vi "test.vi"() -> ()   [LabVIEW 2020]
uses:
  DataSocketCluster external.ctl
panel:
  in  "TimeOut Time (s)":dbl=30.0 format="%.2f"
  out "Response Initialise":string
  out "Response to Load bias parameters":string
  in  "Load bias parameters":bool
  out "Voltage at each step on PJVS curve":dbl[](array[numeric]) format="%#_16g"
  in  "Send AC":bool
  out "Response to SEND AC":string
  out "Return number of steps on PJVS curve":string
  out "Return time interval on PJVS step":string
  out "Frequency calculated (Hz)":dbl=100.0
  in  "Frequency (Hz)":dbl=100.0 format="%#_10g"
  in  "Amplitude (V)":string="1"
  in  "Steps on PJVS curve":u32=100
  out "Calculated time on PJVS step (smallest value is 17)":u32=100
  in  "Name of computer running Bias Source software":string="CZC105BD8M"
  in  "This machine (client)":string="localhost"
  out "error out":errorcluster {"code" format="%.0x"}
  in  "error in (no error)":errorcluster
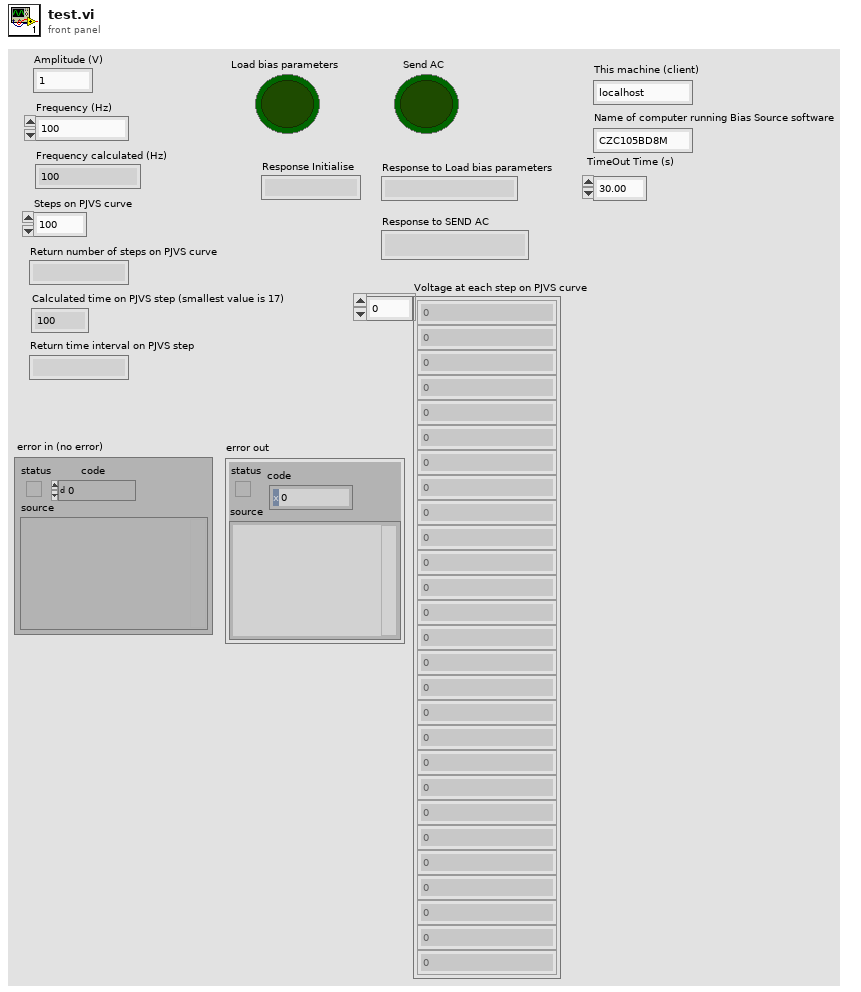
[diagram p1: front panel]
types:
  T1 = typedef "DataSocketCluster external.ctl" = cluster{"Server Machine":string, "Client Machine":string, "Data":string, "TimeStamp":dbl, "Count":i32, "Target Process":string}
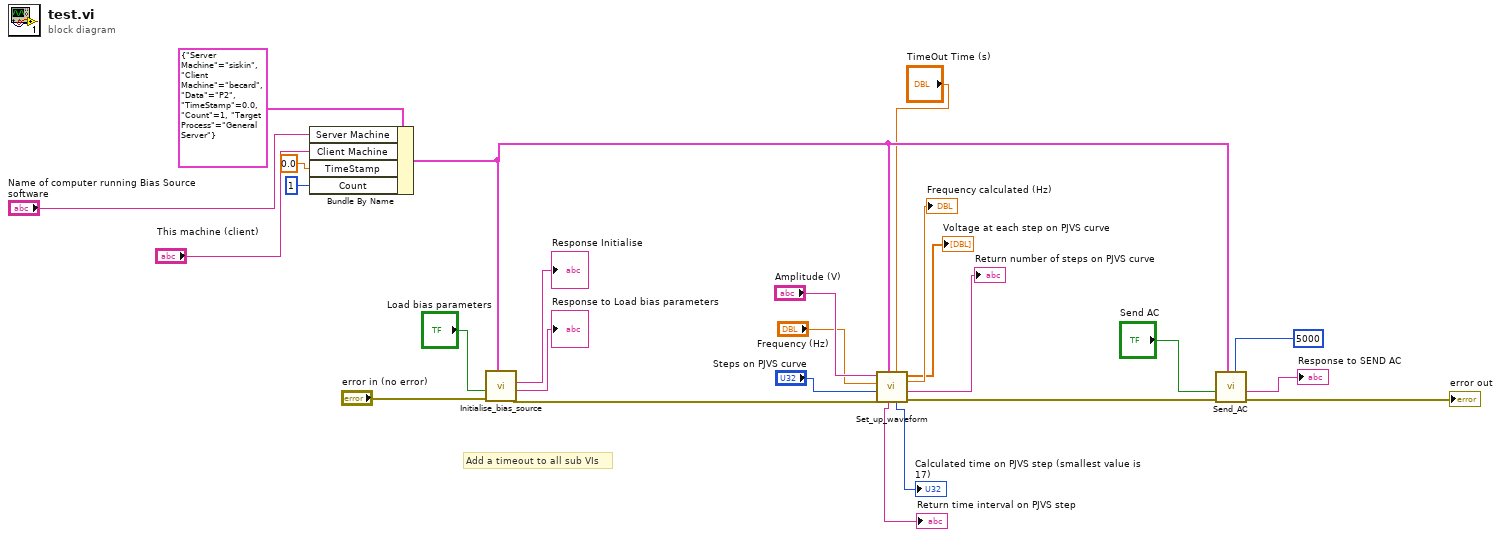
[diagram p0: block diagram]
diagram:
  # "Add a timeout to all sub VIs"
  n1 = Bundle By Name(cluster=T1 {"Server Machine"="siskin", "Client Machine"="becard", "Data"="P2", "TimeStamp"=0.0, "Count"=1, "Target Process"="General Server"} ("DataSocketCluster In"), "Server Machine"="Name of computer running Bias Source software", "Client Machine"="This machine (client)", "TimeStamp"=0.0, "Count"=1) -> (w5:T1)
  n2 = call "Initialise_bias_source.vi"("output cluster"=w5, "error in (no error)"="error in (no error)", "Load bias parameters"="Load bias parameters") -> ("error out"=w16:errorcluster, "Response to Load bias parameters"=→"Response to Load bias parameters":string, "Response Initialise"=→"Response Initialise":string)  [unwired: 6 in]
  n3 = call "Set_up_waveform.vi"("TimeOut Time (s)"="TimeOut Time (s)", "DataSocketCluster In"=w5, "error in (no error)"=w16, "Steps on PJVS curve"="Steps on PJVS curve", "Frequency (Hz)"="Frequency (Hz)", "Amplitude (V)"="Amplitude (V)") -> ("error IO"=w7:errorcluster, "Returned number of steps on PJVS curve"=→"Return number of steps on PJVS curve":string, "Set frequency (Hz)"=→"Frequency calculated (Hz)":dbl, "Voltage at each step on PJVS curve"=→"Voltage at each step on PJVS curve":dbl[], "Calculated time on step (smallest value is 17)"=→"Calculated time on PJVS step (smallest value is 17)":u32, "Returned time interval on each step"=→"Return time interval on PJVS step":string)
  n4 = call "Send_AC.vi"("milliseconds to wait"=u32 5000, 7:w5, "error in (no error)"=w7, 9:"Send AC") -> ("error out"=→"error out":errorcluster, "Response to SEND AC"=→"Response to SEND AC":string)  [unwired: 5 in, 1 out]
